vi "AB_820_850_Project_Destinations.vi"(6 "ProjectPath":path, 7 "action":T3, 8 "error in (no error)":errorcluster, 9 "index":i32, 10 "data in":T2, 11 "buildObject":T1) -> (0 "error out":errorcluster, 1 "index out":i32, 2 "data out":T2, 3 "buildObject out":T1)   [LabVIEW 2020]
doc: "Reads and writes the data to the object property bag."
uses:
  <resource>/Framework/Providers/API/ItemRef.ctl
  <vilib>/AppBuilder/RW_Project/AB_RW_Project_PropBag_Action.ctl
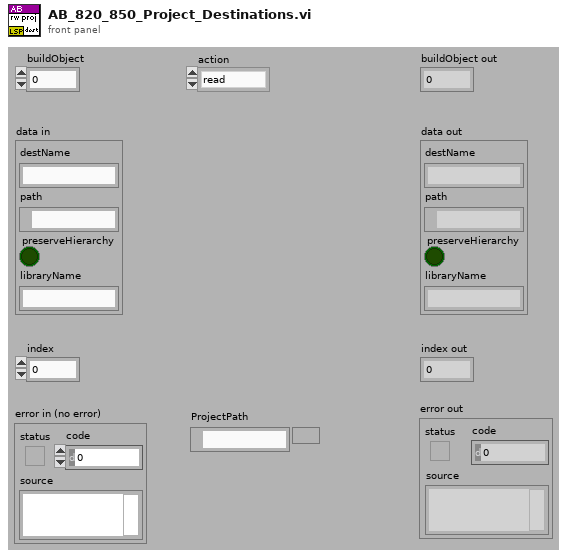
[diagram p1: front panel]
types:
  T1 = typedef "ItemRef.ctl" = u64
  T2 = cluster{"destName":string, "path":path, "preserveHierarchy":bool, "libraryName":string}
  T3 = typedef "AB_RW_Project_PropBag_Action.ctl" = enum16{"read", "write", "clear", "readPrevious", "writePrevious", "clearPrevious"}
  T4 = typedef "AB_820_850_Relative_Path_Type.ctl" = enum16{"<none>", "relativeToCommon", "relativeToAppDir"}
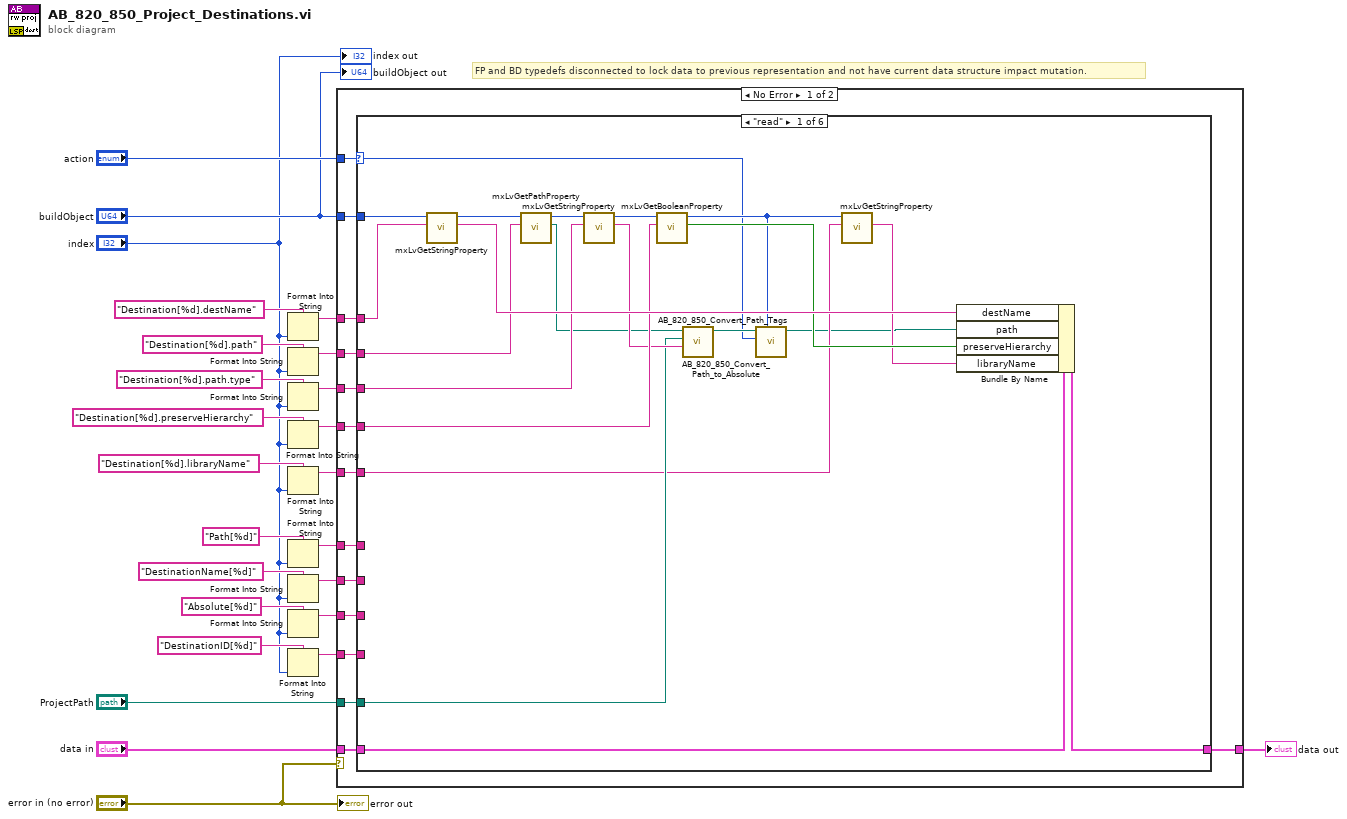
[diagram p0: block diagram]
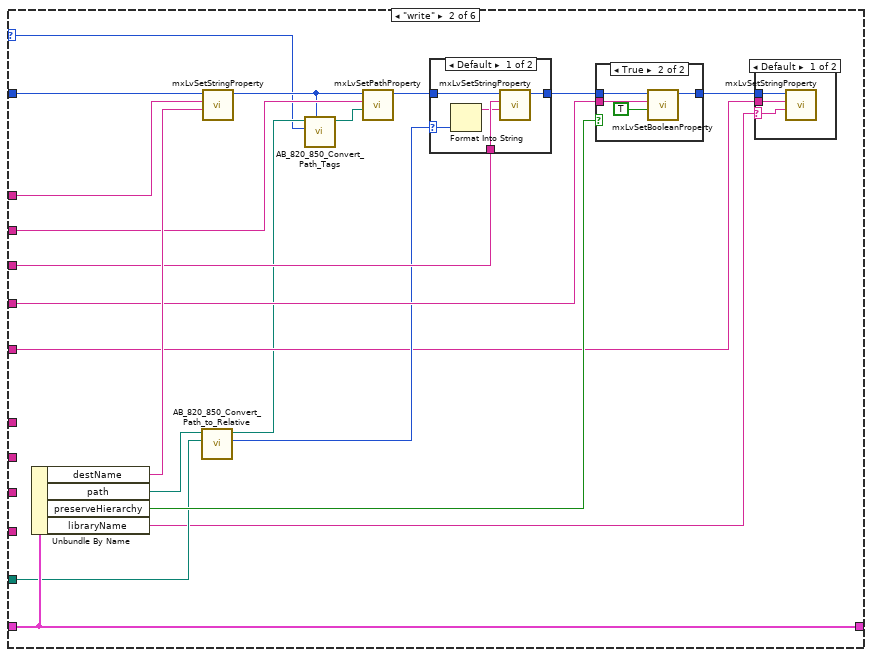
[diagram p2: hidden frame]
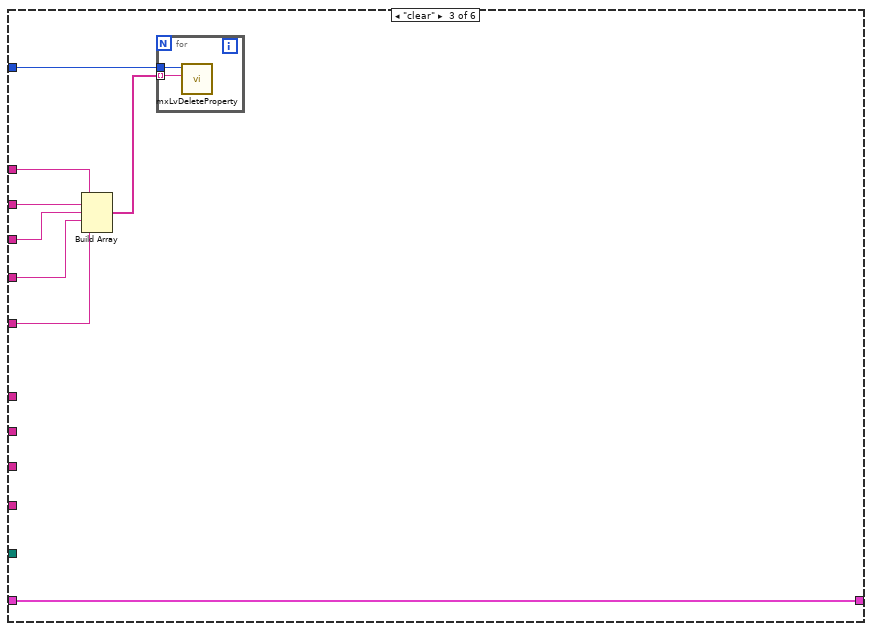
[diagram p6: hidden frame]
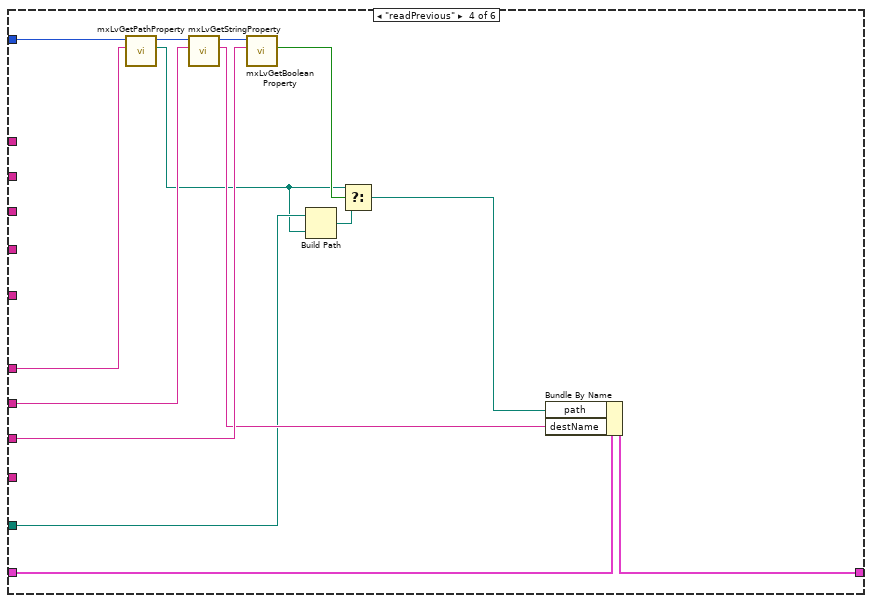
[diagram p7: hidden frame]
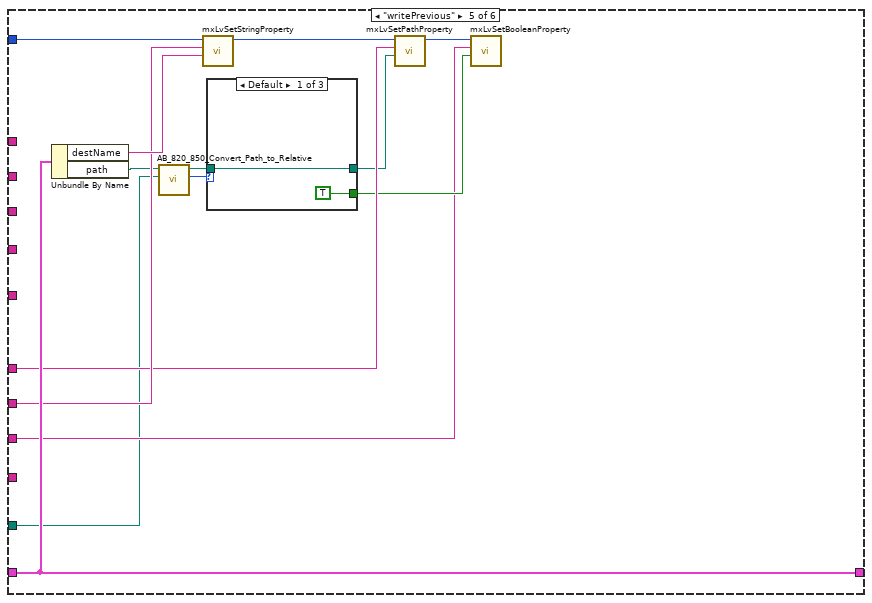
[diagram p8: hidden frame]
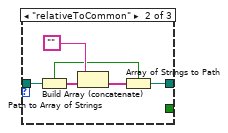
[diagram p9: hidden frame]
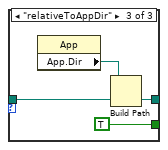
[diagram p10: hidden frame]
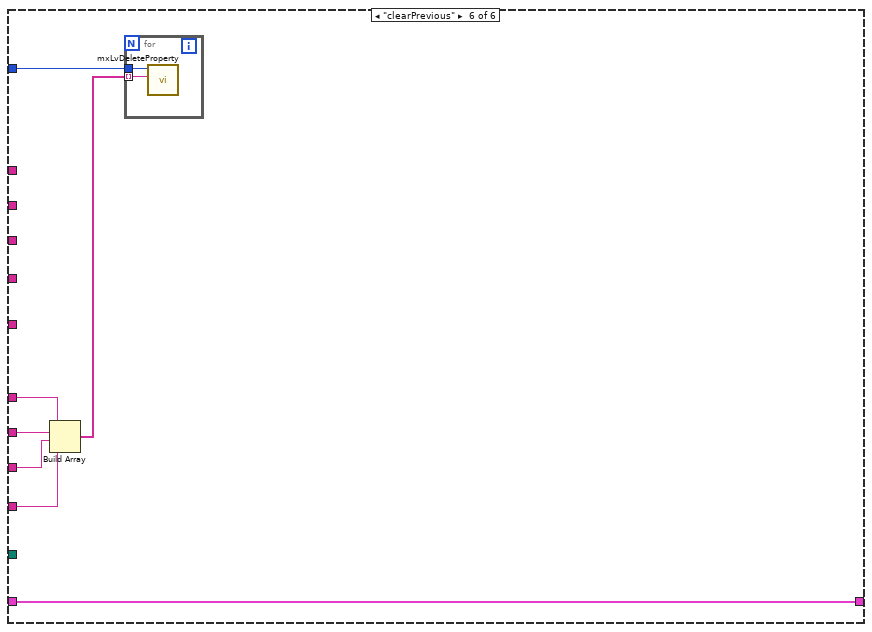
[diagram p11: hidden frame]
diagram:
  # "FP and BD typedefs disconnected to lock data to previous representation and not have current data structure impact mutation."
  n1 = Format Into String(format string="Destination[%d].destName", "index") -> (resulting string=w22:string)  [unwired: 2 in, 1 out]
  n2 = Format Into String(format string="Destination[%d].path", "index") -> (resulting string=w19:string)  [unwired: 2 in, 1 out]
  n3 = Format Into String(format string="Destination[%d].path.type", "index") -> (resulting string=w18:string)  [unwired: 2 in, 1 out]
  n4 = Format Into String(format string="Destination[%d].preserveHierarchy", "index") -> (resulting string=w6:string)  [unwired: 2 in, 1 out]
  n5 = Format Into String(format string="Destination[%d].libraryName", "index") -> (resulting string=w3:string)  [unwired: 2 in, 1 out]
  n6 = Format Into String(format string="Path[%d]", "index") -> (resulting string=w11:string)  [unwired: 2 in, 1 out]
  n7 = Format Into String(format string="DestinationName[%d]", "index") -> (resulting string=w10:string)  [unwired: 2 in, 1 out]
  n8 = Format Into String(format string="Absolute[%d]", "index") -> (resulting string=w9:string)  [unwired: 2 in, 1 out]
  n9 = Format Into String(format string="DestinationID[%d]", "index") -> (resulting string=w5:string)  [unwired: 2 in, 1 out]
  n10 = case shown="No Error" "error in (no error)" {
    tunnel: "action" -> [w39 _]
    tunnel: "data in" -> [w38 w154]
    tunnel: w22 -> [w37 _]
    tunnel: w19 -> [w36 _]
    tunnel: w18 -> [w35 _]
    tunnel: [w34 w154] -> w17
    tunnel: "buildObject" -> [w33 _]
    tunnel: w11 -> [w32 _]
    tunnel: w10 -> [w31 _]
    tunnel: w9 -> [w30 _]
    tunnel: "ProjectPath" -> [w29 _]
    tunnel: w6 -> [w28 _]
    tunnel: w5 -> [w27 _]
    tunnel: w3 -> [w26 _]
    frame No Error {
      n11 = case shown="\"read\"" w39 {
        selector: w39 -> [w40 w61 _ _ _ _]
        tunnel: w33 -> [w60 w79 w98 w115 w131 w150]
        tunnel: w38 -> [w59 w80 w102 w112 w132 w151]
        tunnel: w37 -> [w57 w78 w100 _ _ _]
        tunnel: w36 -> [w53 w76 w101 _ _ _]
        tunnel: w35 -> [w52 w75 w99 _ _ _]
        tunnel: [w56 w80 w102 w111 w132 w151] -> w34
        tunnel: w32 -> [_ _ _ w105 w127 w147]
        tunnel: w31 -> [_ _ _ w114 w128 w148]
        tunnel: w30 -> [_ _ _ w113 w123 w146]
        tunnel: w29 -> [w47 w70 _ w107 w122 _]
        tunnel: w28 -> [w49 w71 w96 _ _ _]
        tunnel: w27 -> [_ _ _ _ _ w145]
        tunnel: w26 -> [w44 w67 w95 _ _ _]
        frame "read" {
          n12 = call <resource>:"mxLvGetStringProperty.vi"("Tag"=w57, "Item"=w60) -> ("Value"=w58:string, "Item"=w54:T1)  [unwired: 7 in, 1 out]
          n13 = call <resource>:"mxLvGetPathProperty.vi"("Tag"=w53, "Item"=w54) -> ("Path"=w46:path, "Item"=w55:T1)  [unwired: 7 in, 1 out]
          n14 = call <resource>:"mxLvGetStringProperty.vi"("Tag"=w52, "Item"=w55) -> ("Value"=w48:string, "Item"=w51:T1)  [unwired: 7 in, 1 out]
          n15 = call <resource>:"mxLvGetBooleanProperty.vi"("Tag"=w49, "Item"=w51) -> ("Value"=w50:bool, "Item"=w43:T1)  [unwired: 7 in, 1 out]
          n16 = call <vilib>:"AB_820_850_Convert_Path_to_Absolute.vi"("relativeType"=w48, "commonPath"=w47, "relativePath"=w46) -> ("absolute path"=w42:path)  [unwired: 7 in, 1 out]
          n17 = call <vilib>:"AB_820_850_Convert_Path_Tags.vi"("buildObject"=w43, "action"=w40, "Path in"=w42) -> ("Path out"=w41:path)  [unwired: 7 in, 1 out]
          n18 = call <resource>:"mxLvGetStringProperty.vi"("Tag"=w44, "Item"=w43) -> ("Value"=w45:string)  [unwired: 7 in, 2 out]
          n19 = Bundle By Name(cluster=w59, "destName"=w58, "path"=w41, "preserveHierarchy"=w50, "libraryName"=w45) -> (w56:T2)
        }
        frame "write" {
          n20 = Unbundle By Name(w80) -> ("destName"=w77:string, "path"=w69:path, "preserveHierarchy"=w72:bool, "libraryName"=w65:string)
          n21 = call <vilib>:"AB_820_850_Convert_Path_to_Relative.vi"("commonPath"=w70, "absolutePath"=w69) -> ("relativeType"=w68:T4, "newPath"=w63:path)  [unwired: 7 in, 1 out]
          n22 = call <resource>:"mxLvSetStringProperty.vi"("Value (\"\")"=w77, "Tag"=w78, "Item"=w79) -> ("Item"=w64:T1)  [unwired: 7 in, 1 out]
          n23 = call <vilib>:"AB_820_850_Convert_Path_Tags.vi"("buildObject"=w64, "action"=w61, "Path in"=w63) -> ("Path out"=w62:path)  [unwired: 7 in, 1 out]
          n24 = call <resource>:"mxLvSetPathProperty.vi"("Path"=w62, "Tag"=w76, "Item"=w64) -> ("Item"=w74:T1)  [unwired: 7 in, 1 out]
          n25 = case shown="Default" w68 {
            selector: w68 -> [w92 _]
            tunnel: w74 -> [w93 w94]
            tunnel: w75 -> [w91 _]
            tunnel: [w89 w94] -> w73
            frame Default {
              n26 = Format Into String(w92) -> (resulting string=w90:string)  [unwired: 3 in, 1 out]
              n27 = call <resource>:"mxLvSetStringProperty.vi"("Value (\"\")"=w90, "Tag"=w91, "Item"=w93) -> ("Item"=w89:T1)  [unwired: 7 in, 1 out]
            }
            frame "relativeToCommon" {
            }
          }
          n28 = case shown="True" w72 {
            tunnel: w73 -> [w84 w88]
            tunnel: w71 -> [_ w87]
            tunnel: [w84 w85] -> w66
            frame False {
            }
            frame True {
              n29 = call <resource>:"mxLvSetBooleanProperty.vi"("Value (F)"=TRUE, "Tag"=w87, "Item"=w88) -> ("Item"=w85:T1)  [unwired: 7 in, 1 out]
            }
          }
          n30 = case shown="Default" w65 {
            selector: w65 -> [w81 _]
            tunnel: w66 -> [w82 _]
            tunnel: w67 -> [w83 _]
            frame Default {
              n31 = call <resource>:"mxLvSetStringProperty.vi"("Value (\"\")"=w81, "Tag"=w83, "Item"=w82) -> ()  [unwired: 7 in, 2 out]
            }
            frame "" {
            }
          }
        }
        frame "clear" {
          n32 = Build Array(w100, w101, w99, w96, w95) -> (w97:string[])
          n33 = for {
            tunnel: w98 -> [w104]
            tunnel: w97 -> [w103] mode=indexing
            n34 = call <resource>:"mxLvDeleteProperty.vi"("Tag"=w103, "Item"=w104) -> ()  [unwired: 8 in, 2 out]
          }
        }
        frame "readPrevious" {
          n35 = call <resource>:"mxLvGetPathProperty.vi"("Tag"=w105, "Item"=w115) -> ("Path"=w106:path, "Item"=w118:T1)  [unwired: 7 in, 1 out]
          n36 = call <resource>:"mxLvGetStringProperty.vi"("Tag"=w114, "Item"=w118) -> ("Value"=w110:string, "Item"=w117:T1)  [unwired: 7 in, 1 out]
          n37 = call <resource>:"mxLvGetBooleanProperty.vi"("Tag"=w113, "Item"=w117) -> ("Value"=w108:bool)  [unwired: 7 in, 2 out]
          n38 = Build Path(base path=w107, name or relative path=w106) -> (appended path=w116:path)
          n39 = Select(t=w106, s=w108, f=w116) -> (s? t:f=w109:path)
          n40 = Bundle By Name(cluster=w112, "path"=w109, "destName"=w110) -> (w111:T2)
        }
        frame "writePrevious" {
          n41 = Unbundle By Name(w132) -> ("destName"=w130:string, "path"=w120:path)
          n42 = call <vilib>:"AB_820_850_Convert_Path_to_Relative.vi"("commonPath"=w122, "absolutePath"=w120) -> ("relativeType"=w121:T4, "newPath"=w119:path)  [unwired: 7 in, 1 out]
          n43 = call <resource>:"mxLvSetStringProperty.vi"("Value (\"\")"=w130, "Tag"=w128, "Item"=w131) -> ("Item"=w129:T1)  [unwired: 7 in, 1 out]
          n44 = case shown="Default" w121 {
            tunnel: w119 -> [w134 w140 w143]
            tunnel: [w134 w135 w142] -> w126
            tunnel: [TRUE _ TRUE] -> w124
            frame Default {
            }
            frame "relativeToCommon" {
              n45 = Path to Array of Strings(0:w140) -> (1:w136:bool, 2:w139:string[])
              n46 = Build Array (concatenate)("", w139) -> (w137:string[])
              n47 = Array of Strings to Path(0:w137, 1:w136) -> (2:w135:path)
            }
            frame "relativeToAppDir" {
              n48 = property class="App"() -> ("App.Dir"=w144:path)  [unwired: 2 in, 2 out]
              n49 = Build Path(base path=w144, name or relative path=w143) -> (appended path=w142:path)
            }
          }
          n50 = call <resource>:"mxLvSetPathProperty.vi"("Path"=w126, "Tag"=w127, "Item"=w129) -> ("Item"=w125:T1)  [unwired: 7 in, 1 out]
          n51 = call <resource>:"mxLvSetBooleanProperty.vi"("Value (F)"=w124, "Tag"=w123, "Item"=w125) -> ()  [unwired: 7 in, 2 out]
        }
        frame "clearPrevious" {
          n52 = Build Array(w147, w148, w146, w145) -> (w149:string[])
          n53 = for {
            tunnel: w150 -> [w153]
            tunnel: w149 -> [w152] mode=indexing
            n54 = call <resource>:"mxLvDeleteProperty.vi"("Tag"=w152, "Item"=w153) -> ()  [unwired: 8 in, 2 out]
          }
        }
      }
    }
    frame Error {
    }
  }
  "data out" <- w17
  "error out" <- "error in (no error)"
  "buildObject out" <- "buildObject"
  "index out" <- "index"
